vi "CAPTH-Seek.vi"(0 "Start atten":dbl, 1 "Navg":i32, 2 "Response":T3={"Averages (3dB steps)"=0, "Time Window (ms)"=1.0, "dt (us)"=5.0, "Grass gain"=18.0, "CRITERION (mV)"=5.0, "CEILING (dB atten)"=8.0, "Use previous"=FALSE, "Save avgs"=FALSE, "Save raw"=FALSE, "Save history"=FALSE, "CEILING (dB SPL)"=6.0} {"CRITERION (mV)" format="%.2f"; "Time Window (ms)" format="%.2f"}, 3 "Max SPL":dbl, 5 "AO channels":u16[](array[numeric]), 7 "suprathreshold?":bool, 9 "Runtime":T2, 11 "error in (no error)":errorcluster, 12 "step size":i32, 13 "dB ref":refnum<vi>, 14 "IPC":T1) -> (4 "End atten":dbl, 6 "abort":bool, 8 "suprathreshold out":bool, 10 "any supra":bool, 15 "error out":errorcluster)   [LabVIEW 2020]
uses:
  Typedefs/CAPTH-Response.ctl
  Typedefs/CAPTH-Runtime.ctl
  Typedefs/CAPTH-IPC.ctl
  Typedefs/CAPTH-Start Data.ctl
  Typedefs/CAPTH-Parameters.ctl
  Typedefs/CAPTH-Stimulus.ctl
  Typedefs/CAPTH-Analysis Message.ctl
  Typedefs/CAPTH-Analysis Action.ctl
  Typedefs/CAPTH-StimCon.ctl
  Typedefs/CAPTH-Analysis Data Properties.ctl
  epl-vi-lib/Utility VIs/Math VIs/dB to Linear (scalar).vi
  epl-vi-lib/PXI DAQ VIs/DAQ Engine VIs/AO Gain and Multiplier VIs/PXI Multipliers to AO Gains (1D).vi
  epl-vi-lib/Utility VIs/Math VIs/interp1.vi
panel:
  out "end (interp)":dbl
  out "Attenuation":dbl(graph)
  out "Peak-to-Peak":dbl(graph)
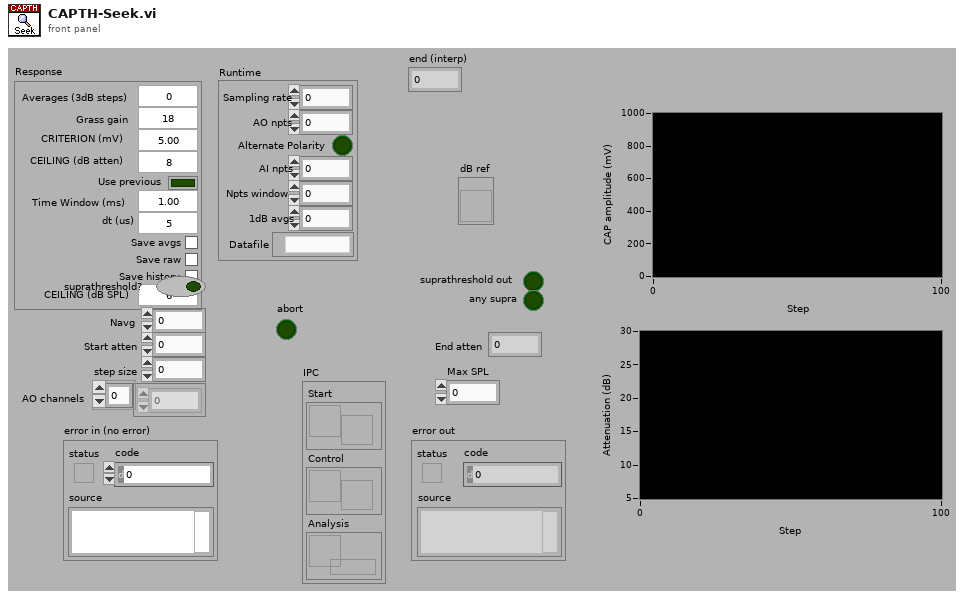
[diagram p1: front panel]
types:
  T1 = typedef "CAPTH-IPC.ctl" = cluster{"Start":refnum<notifier>, "Control":refnum<notifier>, "Analysis":refnum<queue>}
  T2 = typedef "CAPTH-Runtime.ctl" = cluster{"Sampling rate":dbl, "AO npts":i32, "Alternate Polarity":bool, "AI npts":i32, "Npts window":i32, "1dB avgs":i32, "Datafile":path}
  T3 = typedef "CAPTH-Response.ctl" = cluster{"Averages (3dB steps)":i32, "Time Window (ms)":dbl, "dt (us)":dbl, "Grass gain":dbl, "CRITERION (mV)":dbl, "CEILING (dB atten)":dbl, "Use previous":bool, "Save avgs":bool, "Save raw":bool, "Save history":bool, "CEILING (dB SPL)":dbl}
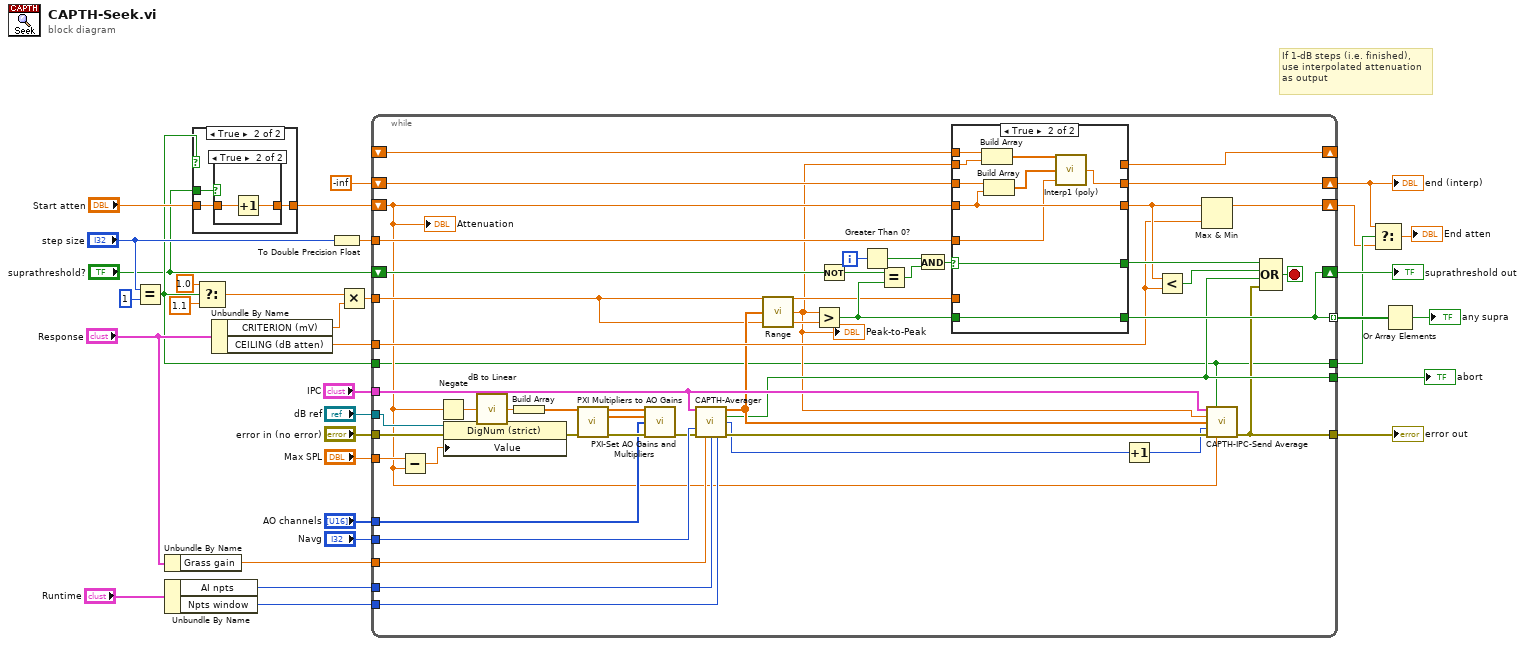
[diagram p0: block diagram]
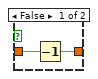
[diagram p3: hidden frame]
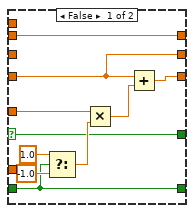
[diagram p4: hidden frame]
diagram:
  # "If 1-dB steps (i.e. finished),\nuse interpolated attenuation\nas output"
  n1 = Equal?(x="step size", y=1 ("x")) -> (x = y?=w7:bool)
  n2 = Unbundle By Name("Response") -> ("Grass gain"=w15:dbl)
  n3 = Unbundle By Name("Runtime") -> ("AI npts"=w13:i32, "Npts window"=w12:i32)
  n4 = case shown="True" w7 {
    tunnel: "Start atten" -> [w35 w36]
    tunnel: [w35 w37] -> w8
    tunnel: "suprathreshold?" -> [_ w38]
    frame False {
    }
    frame True {
      n5 = case shown="True" w38 {
        tunnel: [w39 w41] -> w37
        tunnel: w36 -> [w40 w42]
        frame False {
          n6 = Decrement(x=w40) -> (x-1=w39:dbl)
        }
        frame True {
          n7 = Increment(x=w42) -> (x+1=w41:dbl)
        }
      }
    }
  }
  n8 = Select(t=1.0, s=w7, f=1.1) -> (s? t:f=w26:dbl)
  n9 = Unbundle By Name("Response") -> ("CRITERION (mV)"=w29:dbl, "CEILING (dB atten)"=w20:dbl)
  n10 = To Double Precision Float(number="step size") -> (double precision float=w21:dbl)
  n11 = Multiply(x=w26, y=w29) -> (x*y=w25:dbl)
  n12 = while {
    tunnel: "error in (no error)" -> [w86]
    shift-right: [w61] -> w3
    shift-left: w8 -> [w51]
    tunnel: "AO channels" -> [w65]
    tunnel: w13 -> [w72]
    tunnel: "Navg" -> [w74]
    tunnel: w12 -> [w73]
    tunnel: "dB ref" -> [w85]
    tunnel: [w54] -> w30
    tunnel: w25 -> [w52]
    shift-right: [w63] -> w23
    shift-left: "suprathreshold?" -> [w82]
    tunnel: w21 -> [w78]
    tunnel: w20 -> [w60]
    tunnel: w15 -> [w71]
    tunnel: "Max SPL" -> [w64]
    tunnel: [w63] -> w18 mode=indexing
    tunnel: [w55] -> w11
    tunnel: "IPC" -> [w57]
    tunnel: w7 -> [w45]
    shift-right: [w49] -> w2
    shift-left: -inf -> [w50]
    shift-right: [w48] -> _
    shift-left: _ -> [w46]
    tunnel: [w45] -> w4
    i -> [w81]
    stop <- w53 stop-if-true
    n13 = Subtract(x=w64, y=w51) -> (x-y=w59:dbl)
    n14 = Negate(x=w51) -> (-x=w89:dbl)
    n15 = property class="DigNum (strict)"(reference=w85, error in=w86, "Value"=w59) -> (error out=w84:errorcluster)  [unwired: 1 out]
    n16 = call-poly "dB to Linear.vi"("dB"=w89) -> ("linear"=w88:dbl)
    n17 = Build Array(w88) -> (w87:dbl[])
    n18 = call-poly "PXI Multipliers to AO Gains.vi"("Multipliers in"=w87, "error in (no error)"=w84) -> ("Multipliers out"=w69:dbl[], "Gains"=w68:dbl[], "error out"=w67:errorcluster)  [unwired: 11 in]
    n19 = call "PXI-Set AO Gains and Multipliers.vi"("Multipliers"=w69, "Gains"=w68, "AO Channels"=w65, "error in (no error)"=w67) -> ("error out"=w66:errorcluster)  [unwired: 11 in]
    n20 = call "CAPTH-Averager.vi"("IPC"=w57, "Navg"=w74, "error in (no error)"=w66, "Gain"=w71, "AI samples"=w72, "Window length"=w73) -> ("Neural (uV)"=w56:dbl[], "abort"=w55:bool, "#Tries"=w44:i32, "error out"=w58:errorcluster)  [unwired: 5 in, 1 out]
    n21 = call "Range.vi"("Array"=w56) -> ("Range"=w47:dbl)
    "Peak-to-Peak" <- w47
    n22 = Greater?(x=w47, y=w52) -> (0:w77:bool)
    n23 = Not(x=w82) -> (.not. x?=w83:bool)
    n24 = Greater Than 0?(x=w81) -> (x > 0?=w80:bool)
    n25 = Equal?(x=w83, y=w77) -> (x = y?=w79:bool)
    n26 = And(x=w80, y=w79) -> (x .and. y?=w70:bool)
    n27 = case shown="True" w70 {
      selector: w70 -> [w92 w108]
      tunnel: w51 -> [w91 w105]
      tunnel: w78 -> [w99 w101]
      tunnel: [w94 w105] -> w62
      tunnel: w77 -> [w93 w109]
      tunnel: [w93 w109] -> w63
      tunnel: [w92 w108] -> w76
      tunnel: w52 -> [_ _]
      tunnel: w50 -> [_ w104]
      tunnel: [w91 w100] -> w49
      tunnel: [w90 _] -> w48
      tunnel: w47 -> [w90 w106]
      tunnel: w46 -> [_ w107]
      frame False {
        n28 = Select(t=1.0, s=w93, f=-1.0) -> (s? t:f=w96:dbl)
        n29 = Multiply(x=w99, y=w96) -> (x*y=w95:dbl)
        n30 = Add(x=w91, y=w95) -> (x+y=w94:dbl)
      }
      frame True {
        n31 = Build Array(w107, w106) -> (w103:dbl[])
        n32 = Build Array(w104, w105) -> (w102:dbl[])
        n33 = call-poly "Interp1 (poly).vi"("X"=w103, "Y"=w102, "U"=w101) -> ("V"=w100:dbl)  [unwired: 2 in]
      }
    }
    n34 = Increment(x=w44) -> (x+1=w43:i32)
    n35 = Less?(x=w62, y=w60) -> (x < y?=w75:bool)
    n36 = Max & Min(x=w62, y=w60) -> (max(x,y)=w61:dbl)  [unwired: 1 out]
    n37 = call "CAPTH-IPC-Send Average.vi"("IPC"=w57, "1-dB steps"=w45, "Vp-p"=w47, "Data"=w56, "Ntries"=w43, "error in (no error)"=w58, "Atten"=w51) -> ("error out"=w54:errorcluster)  [unwired: 8 in]
    n38 = Compound Arithmetic op=OR(w76, w75, w55, w54) -> (w53:bool)
    "Attenuation" <- w51
  }
  "error out" <- w30
  "suprathreshold out" <- w23
  "abort" <- w11
  "end (interp)" <- w2
  n39 = Select(t=w2, s=w4, f=w3) -> (s? t:f=→"End atten":dbl)
  n40 = Or Array Elements(Boolean array=w18) -> (logical OR=→"any supra":bool)
